vi "Get filter wheel settings.vi"(6 "Skip pixel":bool) -> (0 "All filter wheel settings":dbl[][](array[numeric]), 1 "Filter intensities":dbl[](array[numeric]), 2 "Filter wheel angles":dbl[](array[numeric]), 3 "Filter wheel numbers":dbl[](array[numeric]), 5 "Filter wheel settings file path":path)   [LabVIEW 2016]
uses:
  <vilib>/Utility/file.llb/Read From Spreadsheet File (DBL).vi
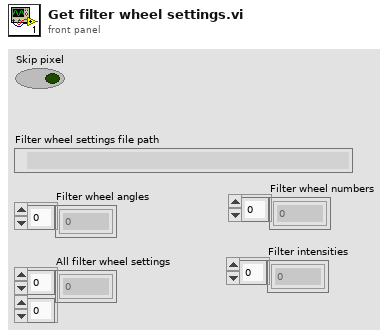
[diagram p1: front panel]
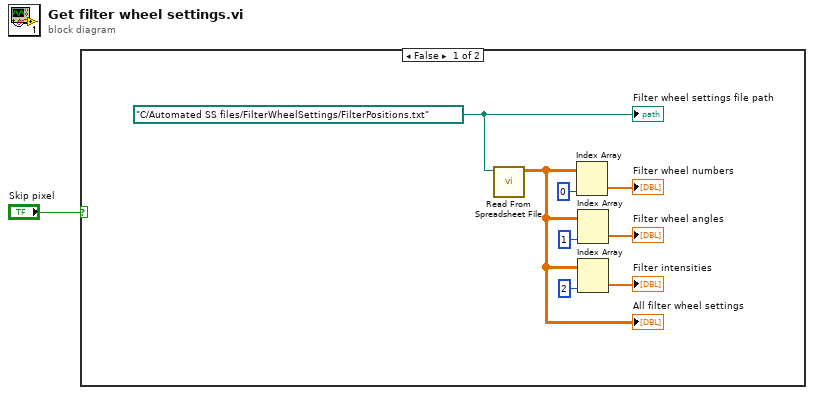
[diagram p0: block diagram]
diagram:
  n1 = case shown="False" "Skip pixel" {
    frame False {
      w9 = path "C:/Automated SS files/FilterWheelSettings/FilterPositions.txt" ("file path (dialog if empty)")
      n2 = call-poly <vilib>:"Read From Spreadsheet File.vi"("file path (dialog if empty)"=w9) -> ("all rows"=w2:dbl[][])  [unwired: 6 in, 4 out]
      "All filter wheel settings" <- w2
      n3 = Index Array(array=w2, index (col)=0 ("disabled index (col)")) -> (element=→"Filter wheel numbers":dbl[])  [unwired: 1 in]
      n4 = Index Array(array=w2, index (col)=1 ("disabled index (col)")) -> (element=→"Filter wheel angles":dbl[])  [unwired: 1 in]
      n5 = Index Array(array=w2, index (col)=2 ("disabled index (col)")) -> (element=→"Filter intensities":dbl[])  [unwired: 1 in]
      "Filter wheel settings file path" <- w9
    }
    frame True {
    }
  }
